vi "SetSubDatDisplayNm.vi"(8 "error in (no error)":errorcluster caption="entrée d'erreur (pas d'erreur)", 10 "SubDatDisplayNm":string[](array[string]), 11 "BaseDevice en entrée":refnum<class "BaseDevice.lvclass">) -> (0 "error out":errorcluster caption="sortie d'erreur", 3 "BaseDevice en sortie":refnum<class "BaseDevice.lvclass">)   [LabVIEW 2019, in "BaseDevice.lvclass"]
uses:
  BaseDevice.lvclass
  BaseDevice.lvclass/BaseDevice.ctl
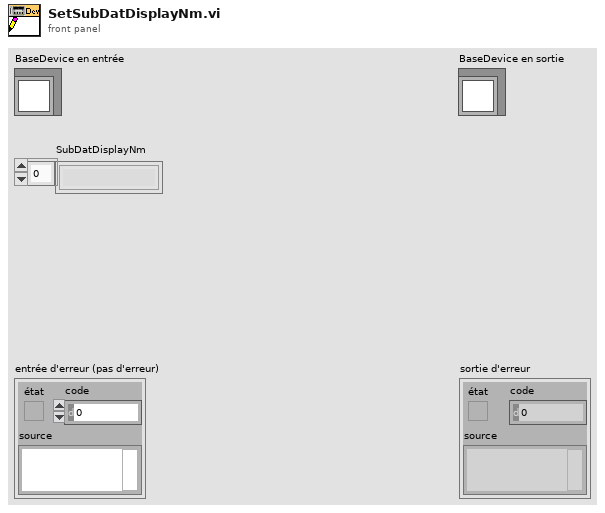
[diagram p1: front panel]
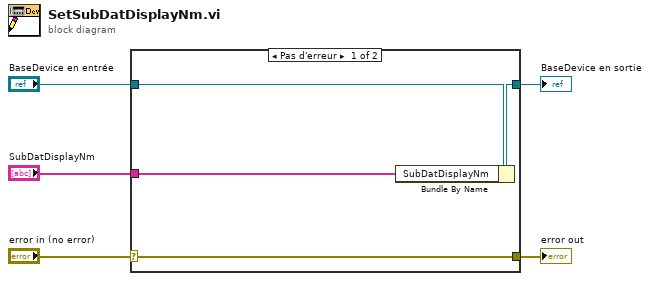
[diagram p0: block diagram]
diagram:
  n1 = case shown="Pas d'erreur" "error in (no error)" {
    selector: "error in (no error)" -> [w9 w10]
    tunnel: [w9 w10] -> w4
    tunnel: [w7 w11] -> w2
    tunnel: "BaseDevice en entrée" -> [w8 w11]
    tunnel: "SubDatDisplayNm" -> [w6 _]
    frame No Error {
      n2 = Bundle By Name(cluster=w8, "SubDatDisplayNm"=w6) -> (w7:refnum<class "BaseDevice.lvclass">)
    }
    frame Error {
    }
  }
  "error out" <- w4
  "BaseDevice en sortie" <- w2
